vi "DisposeCore.vi"(8 "error in (no error)":errorcluster, 11 "RoomWithBomb":refnum<class "RoomWithBomb.lvclass">) -> (0 "error out":errorcluster, 3 "RoomWithBomb":refnum<class "RoomWithBomb.lvclass">)   [LabVIEW 2020, in "RoomWithBomb.lvclass"]
uses:
  RoomWithBomb.lvclass
  Private/TypeDef/privateDataDVR.ctl
  Private/TypeDef/privateData.ctl
  RoomWithBomb.lvclass/RoomWithBomb.ctl
  Room/Room.lvclass
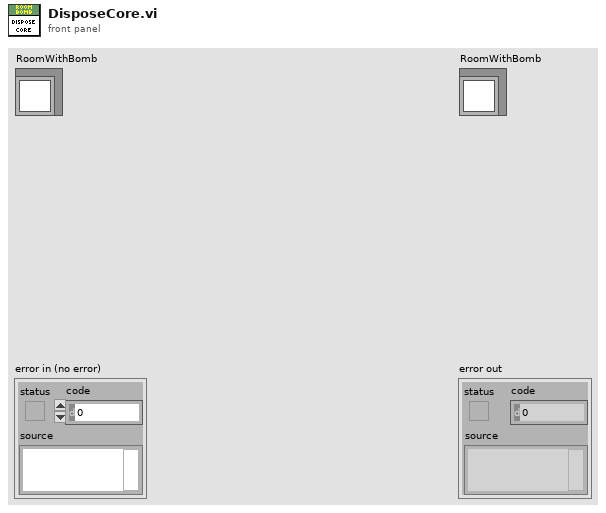
[diagram p1: front panel]
types:
  T1 = typedef "RoomWithBomb.lvclass/privateDataDVR.ctl" = refnum<data-value>
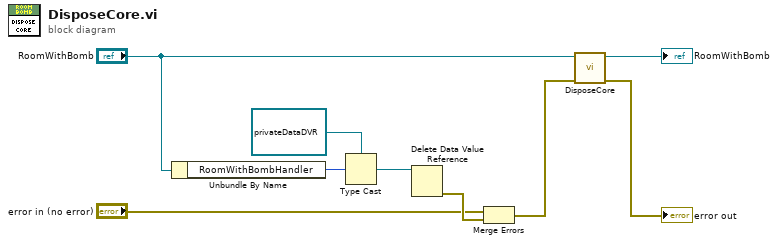
[diagram p0: block diagram]
diagram:
  n1 = Unbundle By Name("RoomWithBomb") -> ("RoomWithBombHandler"=w8:u32)
  n2 = Type Cast(type=T1 refnum ("privateDataDVR"), x=w8) -> (*(type *) &x=w9:T1)
  n3 = Delete Data Value Reference(data value reference=w9) -> (error out=w7:errorcluster)  [unwired: 1 in, 1 out]
  n4 = Merge Errors("error in (no error)", w7) -> (w2:errorcluster)
  n5 = call-parent "DisposeCore.vi"("error in (no error)"=w2, "Room"="RoomWithBomb") -> ("error out"=→"error out":errorcluster, "Room"=→"RoomWithBomb":refnum<class "RoomWithBomb.lvclass">)  [unwired: 8 in]
